vi "Set Segmenting Specification (Time).vi"(5 "Segment File on Trigger (T)":bool=TRUE, 7 "Max Instances (-1: Infinite)":i32=-1, 8 "error in (no error)":errorcluster, 10 "Time Limit":dbl, 11 "Data Logging Specification Ref in":T1) -> (0 "error out":errorcluster, 3 "Data Logging Specification Ref out":T1)   [LabVIEW 2020, in "NI_VS Data Logging API.lvlib"]
doc: "Specifies how to segment the log files created during the data logging session. You can segment log files according to time or size limits, or when a start trigger occurs. When the segmenting condition is met, this VI saves and closes the current log file and continues logging data in a new file.\n\nSelect the Default instance of this VI if you do not want to segment log files based on time or size, but do want the option to segment on a start trigger.\n\nYou must manually select the polymorphic instance to use."
uses:
  <vilib>/NI VeriStand/Execution/DataLogging/NI_VS Data Logging API.lvlib
  <vilib>/NI VeriStand/Execution/DataLogging/DataLoggingSpecification Ref.ctl
  NationalInstruments.VeriStand.ClientAPI
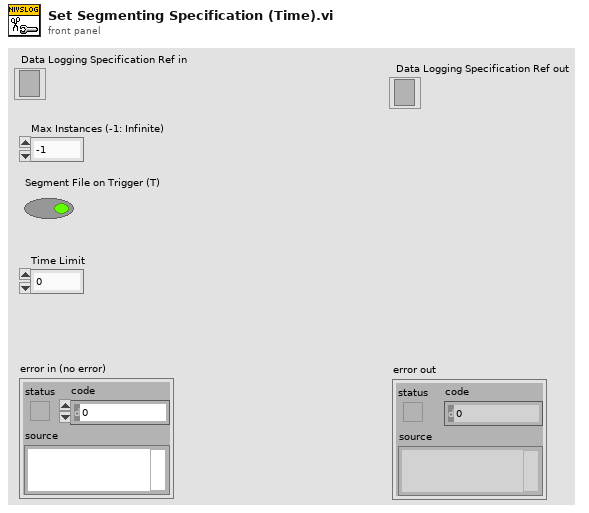
[diagram p1: front panel]
types:
  T1 = typedef "NI_VS Data Logging API.lvlib/DataLoggingSpecification Ref.ctl" = refnum<k24>
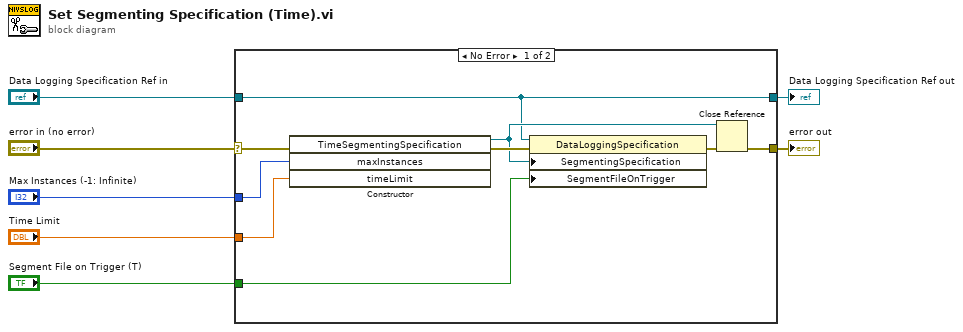
[diagram p0: block diagram]
diagram:
  n1 = case shown="No Error" "error in (no error)" {
    selector: "error in (no error)" -> [w16 w18]
    tunnel: [w12 w18] -> w6
    tunnel: [w10 w17] -> w5
    tunnel: "Data Logging Specification Ref in" -> [w10 w17]
    tunnel: "Max Instances (-1: Infinite)" -> [w15 _]
    tunnel: "Segment File on Trigger (T)" -> [w9 _]
    tunnel: "Time Limit" -> [w8 _]
    frame No Error {
      n2 = constructor class="TimeSegmentingSpecification"(error in=w16, "maxInstances"=w15, "timeLimit"=w8) -> (reference out=w11:refnum<k24>, error out=w14:errorcluster)  [unwired: 2 in, 3 out]
      n3 = property class="DataLoggingSpecification"(reference=w10, error in=w14, "SegmentingSpecification"=w11, "SegmentFileOnTrigger"=w9) -> (error out=w13:errorcluster)  [unwired: 1 out]
      n4 = Close Reference(reference=w11, error in (no error)=w13) -> (error out=w12:errorcluster)
    }
    frame Error {
    }
  }
  "error out" <- w6
  "Data Logging Specification Ref out" <- w5
